vi "Match Time.vi"(8 "error in (no error)":errorcluster, 9 "Length of Appended String Characters (0)":u32, 10 "Control Code":u8(ring) items=["Adjust mode on", "Time request", "Adjust mode off"], 11 "VISA resource name":refnum<visa-resource-name>) -> (0 "error out":errorcluster, 2 "Time":u32, 3 "VISA resource name out":refnum<visa-resource-name>)   [LabVIEW 2011, in "Hokuyo URG Series.lvlib"]
doc: "This command is used to adjust (match) the host and sensor time. Sensor should be switched to adjust mode before requesting its time and mode should be switched off after the adjustment. When the sensor is in adjustment mode laser is switched off and it will not accept any other commands unless the mode is terminated. Before using the Acquire Data command, the laser must be turned back on by using the \"Configure Laser Power\" VI.\n\nSending multiple Match Time Commands with different string lengths and comparing the time can estimate average data transmission time between sensor and host."
uses:
  Hokuyo URG Series.lvlib
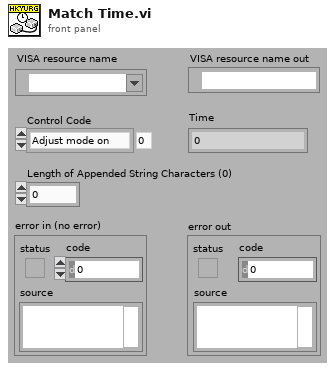
[diagram p1: front panel]
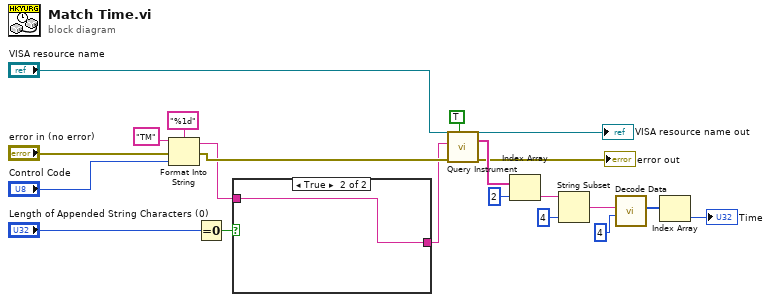
[diagram p0: block diagram]
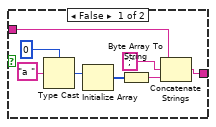
[diagram p2: hidden frame]
diagram:
  n1 = Format Into String(format string="%1d", initial string="TM" ("command"), error in="error in (no error)", "Control Code") -> (resulting string=w6:string, error out=w19:errorcluster)
  n2 = Equal To 0?(x="Length of Appended String Characters (0)") -> (x = 0?=w7:bool)
  n3 = case shown="True" w7 {
    tunnel: [w24 w30] -> w5
    tunnel: w6 -> [w22 w30]
    frame False {
      n4 = Type Cast(type=u8 0, x="a ") -> (*(type *) &x=w29:u8)
      n5 = Initialize Array(w29) -> (w28:u8[])  [unwired: 1 in]
      n6 = Byte Array To String(unsigned byte array=w28) -> (string=w25:string)
      n7 = Concatenate Strings(w22, ";" ("string"), w25) -> (w24:string)
    }
    frame True {
    }
  }
  n8 = call "Query Instrument.vi"("Error Query (Enabled)"=TRUE, "error in"=w19, "Command"=w5, "VISA Resource Name"="VISA resource name") -> ("error out"=→"error out":errorcluster, "Response Strings"=w15:string[], "VISA Resource Name Out"=→"VISA resource name out":refnum<visa-resource-name>)  [unwired: 5 in]
  n9 = Index Array(array=w15, index=2) -> (element=w13:string)
  n10 = String Subset(string=w13, length (rest)=4 ("length (rest)")) -> (substring=w4:string)  [unwired: 1 in]
  n11 = call "Decode Data.vi"("n character encoding"=u32 4, "Input Buffer"=w4) -> ("Decoded Measurements"=w2:i32[])  [unwired: 8 in, 1 out]
  n12 = Index Array(array=w2) -> (element=→"Time":i32)  [unwired: 1 in]
